vi "认识簇.vi"() -> ()   [LabVIEW 2018]
panel:
  out "字符串":string
  in  "簇":cluster{"数值":dbl, "时间标识":timestamp, "布尔":bool}
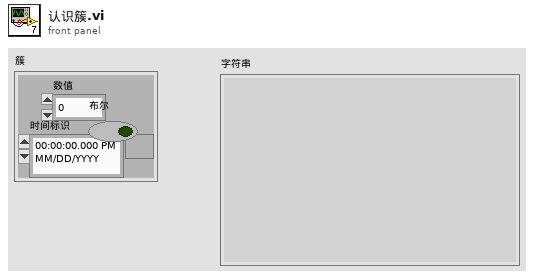
[diagram p1: front panel]
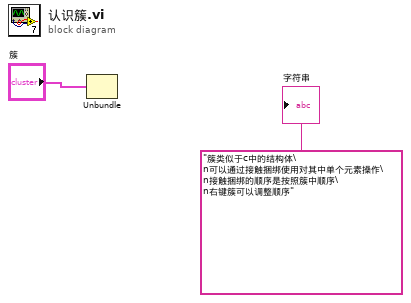
[diagram p0: block diagram]
diagram:
  n1 = Unbundle("簇") -> ()  [unwired: 3 out]
  "字符串" <- "簇类似于c中的结构体\n可以通过接触捆绑使用对其中单个元素操作\n接触捆绑的顺序是按照簇中顺序\n右键簇可以调整顺序"
